vi "Build string_ColumnsName=ColumnsValue_Set.vi"(9 "ColumnsValue":string[](array[string]), 11 "ColumnsNameList":string[](array[string])) -> (2 "Total ColumnName='ColumnValue' String":string)   [LabVIEW 2021, in "DataBase_SQL.lvclass"]
doc: "UPDATE\ntable_name\nSET\ncolumn1=value1,column2=value2,...\nWHERE\nsome_column=some_value\n\nbuild the columnName= 'ColumnValue' string. include all the column names and column values.\n2014-10-31 14:19:04\n蒋松\n\nProjectNum='T0123456',WorkOrder='11M',WO_Description='',LaborRateID='1',MechanicalEngineer='323',ControlEngineer='532',ProjectManager='234',MechanicalAssembly='34',ControlAssembly='234',MechanicalPurchase='34055.7',ControlPurchase='670720.15'"
uses:
  <userlib>/John_Lib/DataBase/DataBase_SQL/DataBase_SQL.lvclass
  <userlib>/John_Lib/DataBase/DataBase_SQL/DataBase_SQL.lvclass/DataBase_SQL.ctl
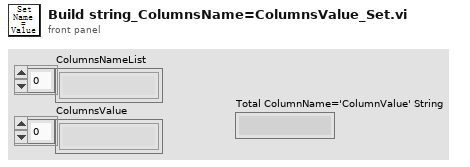
[diagram p1: front panel]
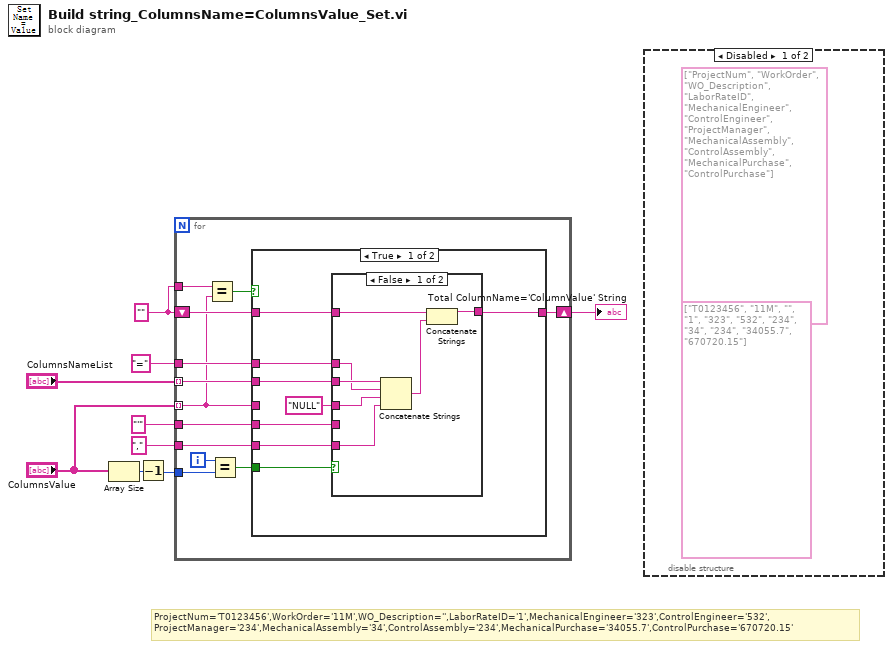
[diagram p0: block diagram]
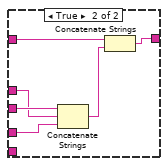
[diagram p3: hidden frame]
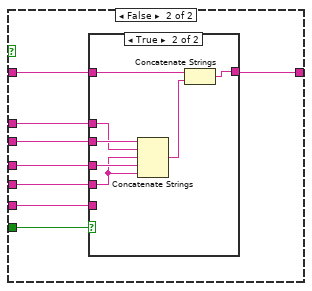
[diagram p4: hidden frame]
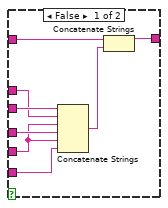
[diagram p5: hidden frame]
diagram:
  w1 = "" ("string")
  # "ProjectNum='T0123456',WorkOrder='11M',WO_Description='',LaborRateID='1',MechanicalEngineer='323',ControlEngineer='532',\nProjectManager='234',MechanicalAssembly='34',ControlAssembly='234',MechanicalPurchase='34055.7',ControlPurchase='670720.15'"
  n1 = Array Size(array="ColumnsValue") -> (size(s)=w6:i32)
  n2 = Decrement(x=w6) -> (x-1=w5:i32)
  n3 = for {
    tunnel: "ColumnsNameList" -> [w12] mode=indexing
    tunnel: "ColumnsValue" -> [w10] mode=indexing
    shift-right: [w15] -> w4
    shift-left: w1 -> [w14]
    tunnel: "=" ("string") -> [w21]
    tunnel: "'" ("string") -> [w20]
    tunnel: "," ("string") -> [w19]
    tunnel: w5 -> [w17]
    tunnel: w1 -> [w13]
    i -> [w18]
    n4 = Equal?(x=w13, y=w10) -> (x = y?=w11:bool)
    n5 = Equal?(x=w18, y=w17) -> (x = y?=w16:bool)
    n6 = case shown="True" w11 {
      tunnel: w12 -> [w29 w50]
      tunnel: w10 -> [_ w49]
      tunnel: w21 -> [w28 w48]
      tunnel: w20 -> [w27 w47]
      tunnel: w19 -> [w26 w46]
      tunnel: w16 -> [w25 w45]
      tunnel: w14 -> [w24 w44]
      tunnel: [w23 w43] -> w15
      frame True {
        n7 = case shown="False" w25 {
          tunnel: w29 -> [w36 w42]
          tunnel: "NULL" ("string") -> [w35 w41]
          tunnel: w28 -> [w34 w40]
          tunnel: w27 -> [_ _]
          tunnel: w26 -> [w33 _]
          tunnel: w24 -> [w32 w39]
          tunnel: [w31 w37] -> w23
          frame False {
            n8 = Concatenate Strings(w36, w34, w35, w33) -> (w30:string)
            n9 = Concatenate Strings(w32, w30) -> (w31:string)
          }
          frame True {
            n10 = Concatenate Strings(w42, w40, w41) -> (w38:string)
            n11 = Concatenate Strings(w39, w38) -> (w37:string)
          }
        }
      }
      frame False {
        n12 = case shown="True" w45 {
          tunnel: w50 -> [w58 w65]
          tunnel: w49 -> [w57 w64]
          tunnel: w48 -> [w56 w63]
          tunnel: w47 -> [w55 w62]
          tunnel: w46 -> [w54 _]
          tunnel: w44 -> [w53 w61]
          tunnel: [w52 w59] -> w43
          frame False {
            n13 = Concatenate Strings(w58, w56, w55, w57, w55, w54) -> (w51:string)
            n14 = Concatenate Strings(w53, w51) -> (w52:string)
          }
          frame True {
            n15 = Concatenate Strings(w65, w63, w62, w64, w62) -> (w60:string)
            n16 = Concatenate Strings(w61, w60) -> (w59:string)
          }
        }
      }
    }
  }
  "Total ColumnName='ColumnValue' String" <- w4
  n17 = disable-structure shown="Disabled" {
    frame Disabled {
      (unwired) string[] ["T0123456", "11M", "", "1", "323", "532", "234", "34", "234", "34055.7", "670720.15"] ("Valid 2D Array 2")
      (unwired) string[] ["ProjectNum", "WorkOrder", "WO_Description", "LaborRateID", "MechanicalEngineer", "ControlEngineer", "ProjectManager", "MechanicalAssembly", "ControlAssembly", "MechanicalPurchase", "ControlPurchase"] ("ColunmsList")
    }
    frame Enabled {
    }
  }
